vi "getStringValue.vi"(8 "error in (no error)":errorcluster, 11 "xmlNode.lvclass in":refnum<class "xmlNode.lvclass">) -> (0 "error out":errorcluster, 2 "stringValue":string, 3 "xmlNode.lvclass out":refnum<class "xmlNode.lvclass">)   [LabVIEW 2009, in "Tools.lvlib" / "xml.lvlib" / "xmlNode.lvclass"]
doc: "Gets the String value of an xml node\ni.e. Gets \"value\" in this example\n\n<xml node> \"value\" </xml node>"
uses:
  xmlNode.lvclass
  xmlNode.lvclass/xmlNode.ctl
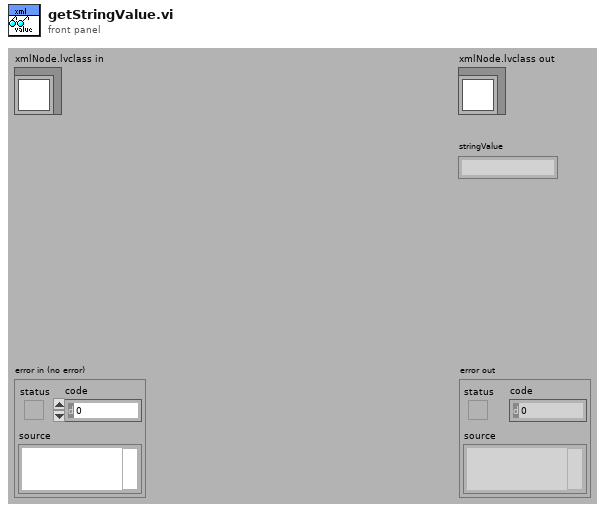
[diagram p1: front panel]
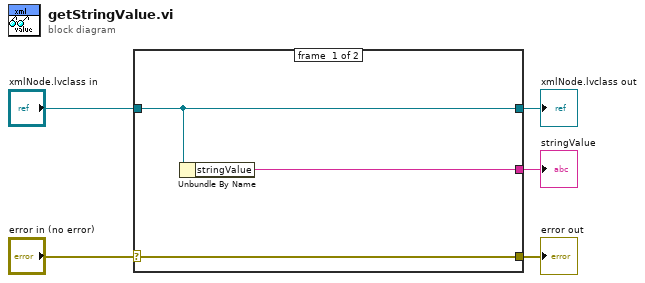
[diagram p0: block diagram]
diagram:
  n1 = case shown="No Error" "error in (no error)" {
    selector: "error in (no error)" -> [w8 w9]
    tunnel: [w8 w9] -> w4
    tunnel: [w7 w10] -> w2
    tunnel: "xmlNode.lvclass in" -> [w7 w10]
    tunnel: [w6 _] -> w1
    frame #0 {
      n2 = Unbundle By Name(w7) -> ("stringValue"=w6:string)
    }
    frame #1 {
    }
  }
  "error out" <- w4
  "xmlNode.lvclass out" <- w2
  "stringValue" <- w1
